vi "On Key Down Event.vi"(6 "Key Event Data in":T1, 8 "error in (no error)":errorcluster, 10 "ScanCode":i16, 11 "App in":refnum<class "App.lvclass">) -> (0 "error out":errorcluster, 2 "Discard":bool, 3 "App out":refnum<class "App.lvclass">, 4 "Key Event Data Out":T1)   [LabVIEW 2020, in "AR Example.lvlib" / "App.lvclass"]
uses:
  App.lvclass
  Key Event Data.ctl
  <vilib>/event_ctls.llb/eventvkey.ctl
  App.lvclass/App.ctl
  UI/UI.lvclass
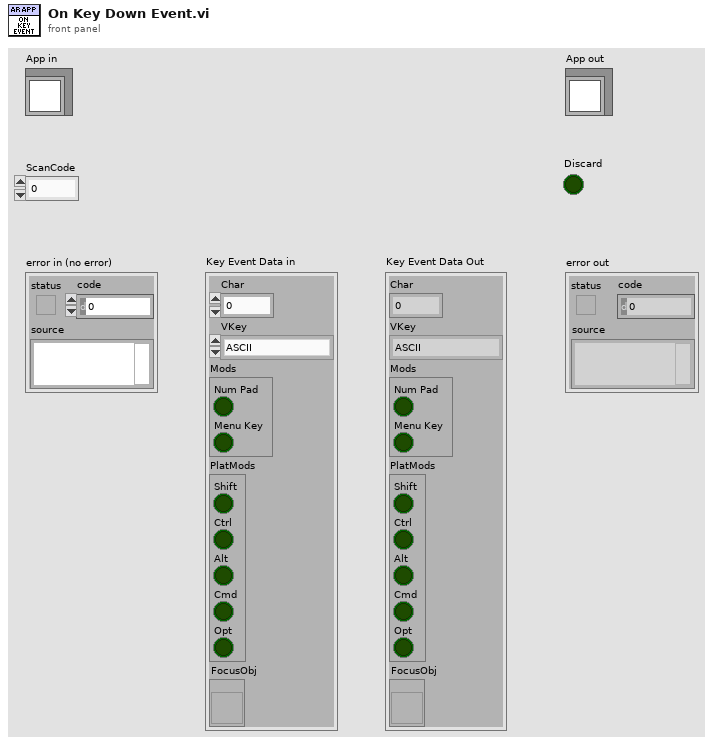
[diagram p1: front panel]
types:
  T1 = typedef "AR Example.lvlib/App.lvclass/Key Event Data.ctl" = cluster{"Char":i16, "VKey":T2, "Mods":cluster{"Num Pad":bool, "Menu Key":bool}, "PlatMods":cluster{"Shift":bool, "Ctrl":bool, "Alt":bool, "Cmd":bool, "Opt":bool}, "FocusObj":refnum<vi>}
  T2 = typedef "eventvkey.ctl" = enum16{"ASCII", "Enter", "Return", "Shift", "Ctrl", "Alt", "Cmd", "Opt", "Caps", "NumLock", "Clear", "Break", "Up", "Down", "Left", "Right", "Insert", "Delete", "Home", "End", "PageUp", "PageDown", "Escape", "Help", "Pause", "ScrollLock", "F1", "F2", "F3", "F4", "F5", "F6", "F7", "F8", "F9", "F10", "F11", "F12", "F13", "F14", "F15", "F16", "F17", "F18", "F19", "F20", "F21", "F22", "F23", "F24", "Play", "VolumeUp", "VolumeDown", "Mute", "Two Byte Char"}
  T3 = typedef "AR Example.lvlib/App.lvclass/Timeout Action.ctl" = enum16{"None", "Setup Camera Action", "Camera Calibration Action"}
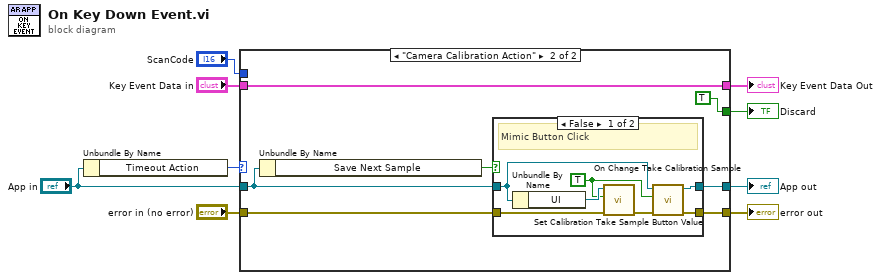
[diagram p0: block diagram]
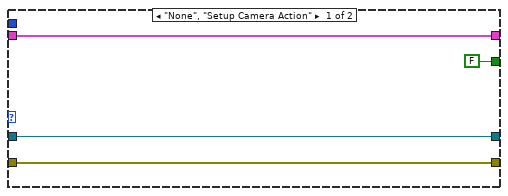
[diagram p2: hidden frame]
diagram:
  n1 = Unbundle By Name("App in") -> ("Timeout Action"=w9:T3)
  n2 = case shown="\"Camera Calibration Action\"" w9 {
    tunnel: "error in (no error)" -> [w12 w14]
    tunnel: [w12 w15] -> w7
    tunnel: "App in" -> [w13 w16]
    tunnel: [w13 w17] -> w5
    tunnel: [w11 w20] -> w4
    tunnel: "Key Event Data in" -> [w11 w20]
    tunnel: [FALSE ("Discard") TRUE ("Discard")] -> w2
    tunnel: "ScanCode" -> [_ _]
    frame "None", "Setup Camera Action" {
    }
    frame "Camera Calibration Action" {
      n3 = Unbundle By Name(w16) -> ("Save Next Sample"=w18:bool)
      n4 = case shown="False" w18 {
        tunnel: [w25 w29] -> w17
        tunnel: w16 -> [w24 w29]
        tunnel: [w26 w28] -> w15
        tunnel: w14 -> [w27 w28]
        frame False {
          w21 = TRUE ("Value")
          # "Mimic Button Click"
          n5 = Unbundle By Name(w24) -> ("UI"=w22:refnum<class "UI.lvclass">)
          n6 = call-dynamic "Set Calibration Take Sample Button Value.vi"("error in (no error)"=w27, "Value"=w21, "UI in"=w22) -> ("error out"=w23:errorcluster)  [unwired: 8 in]
          n7 = call "On Change Take Calibration Sample.vi"("error in (no error)"=w23, "Value"=w21, "App in"=w24) -> ("error out"=w26:errorcluster, "App out"=w25:refnum<class "App.lvclass">)  [unwired: 7 in]
        }
        frame True {
          # "Already Set"
        }
      }
    }
  }
  "error out" <- w7
  "App out" <- w5
  "Key Event Data Out" <- w4
  "Discard" <- w2
